vi "Periodic Tasks.vi"(8 "error in":errorcluster) -> ()   [LabVIEW 2017]
doc: "This VI runs in parallel to other tasks. It can contain as many user-defined periodic loops as you need. These can carry out PID or other sorts of timed response."
uses:
  Robot Global Data.vi
  <vilib>/Rock Robotics/WPI/ThirdParty/Phoenix-LabVIEW/Motor Controller/Controls/CTRE_Phoenix_MotorControl_ControlMode.ctl
  <vilib>/Rock Robotics/WPI/ThirdParty/Sensors/navX/_TypeDefs/FRIC_navX_DeviceNumbersTypeDef.ctl
  <vilib>/addons/control/pid/NI_PID_pid.lvlib
  <vilib>/Rock Robotics/WPI/ThirdParty/Phoenix-LabVIEW/Motor Controller/Get/CTRE_Phoenix_MotorController_GetQuadratureData.vi
  <vilib>/Rock Robotics/WPI/Solenoid/WPI_SolenoidValue.ctl
  Robust CSV/Robust CSV.lvlib
  Robust CSV/Write CSV File_2D.vi
  <vilib>/addons/control/pid/pid.llb/PID (DBL).vi
  <vilib>/Rock Robotics/WPI/Solenoid/WPI_SolenoidSetEnum.vi
panel:
  out "Loop Time":u32
  out "Right":cluster{dbl, i32}(graph)
  out "Left":T1(graph)
  out "clawUp":bool
  out "clawOpen":bool
  out "clawOut":bool
  out "clawIn":bool
  out "2slide":dbl
  out "1Sslide":dbl
  out "MotionProfilePos_Right":dbl
  out "MotionProfilePos_Left":dbl
  out "Right Pos Acutal":i32
  out "Left Pos Acutal":i32
  out "drive speed array":dbl[](array[numeric])
  out "Right Drive Speed":dbl
  out "Left Drive Speed":dbl
  out "output array":dbl[][](array[numeric])
  out "left 2":i32
  out "right 2":i32
  out "Yaw":dbl
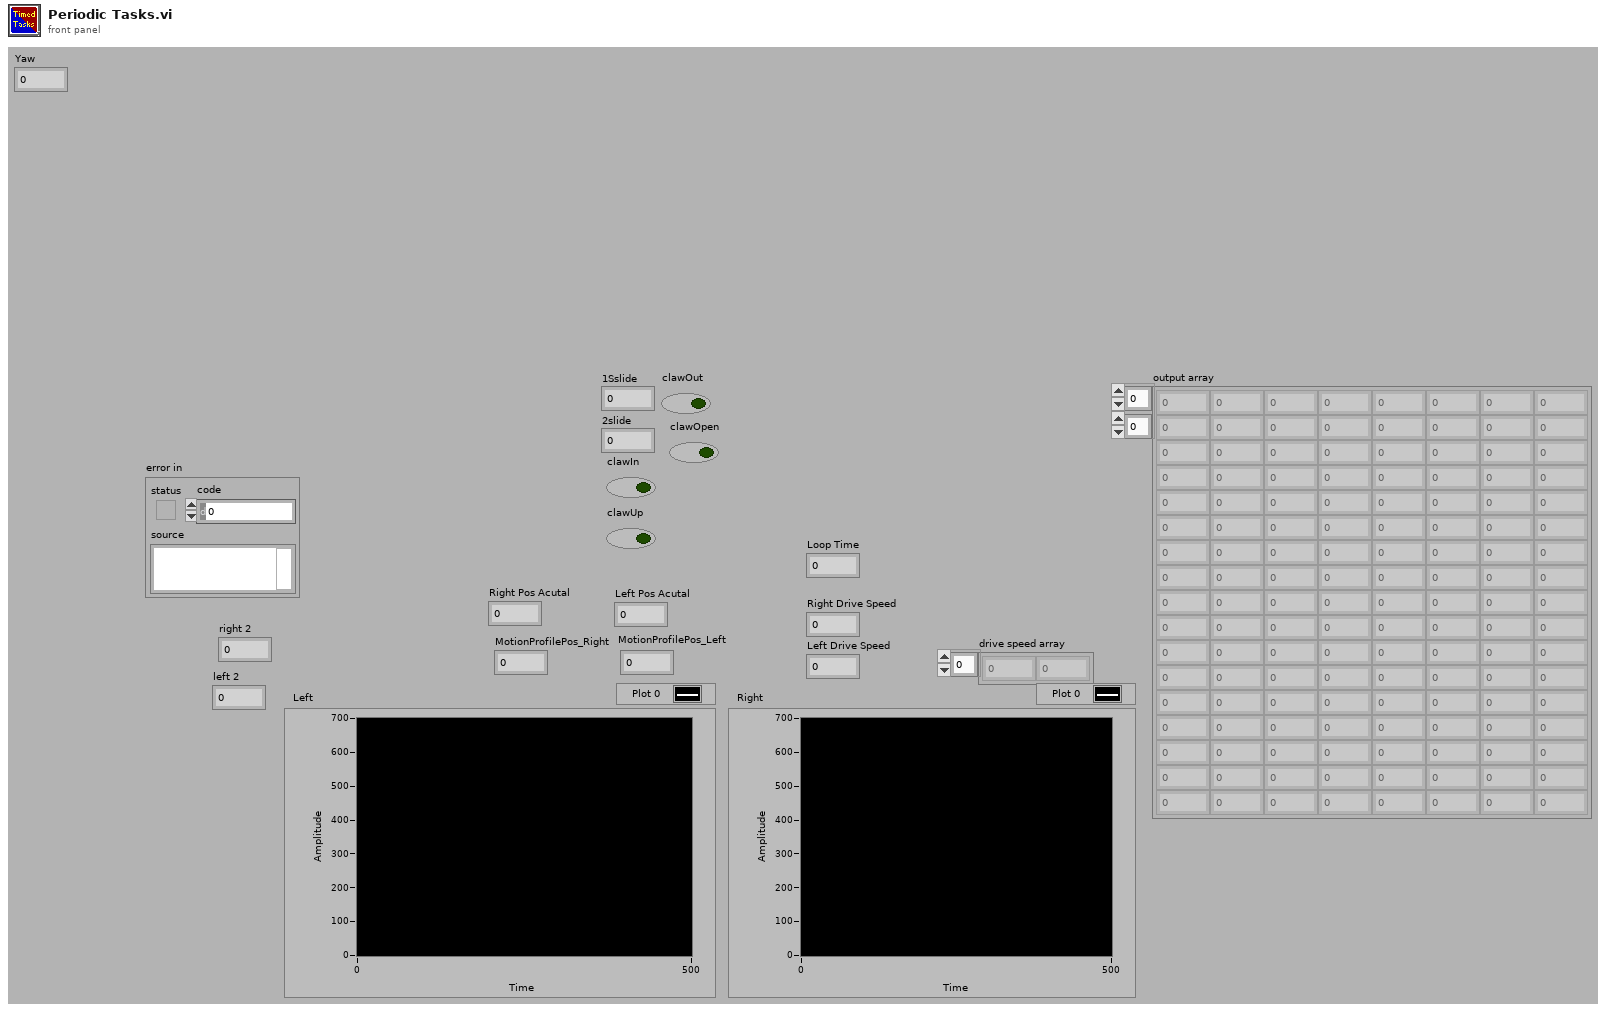
[diagram p1: front panel]
types:
  T1 = cluster{"MotionProfileVel_Right":dbl, "Quadrature Velocity":i32}
  T2 = typedef "WPI_MotorControlDeviceRef.ctl" = cluster{"DeviceStatus":errorcluster, "Type":T3, "PWM":cluster{"PWM Channel":T4, "DeadBand":T5}, "CAN":cluster{"Device Number":u8, "SetOutput VI Ref":variant, "GetOutput VI Ref":variant, "Enable VI Ref":variant, "Disable VI Ref":variant, "Data":variant}, "Invert":bool, "DIO PWM":cluster{"PWM \"Enable\" Channel":T4, "DIOChannel":T6, "PWM Rate":dbl}}
  T3 = typedef "WPI_MotorControlType.ctl" = enum16{"PWM", "CAN", "DIO PWM"}
  T4 = typedef "FPGA_DIOPWMChannel.ctl" = enum8{"PWM 0", "PWM 1", "PWM 2", "PWM 3", "PWM 4", "PWM 5", "PWM 6", "PWM 7", "PWM 8", "PWM 9", "PWM MXP 0", "PWM MXP 1", "PWM MXP 2", "PWM MXP 3", "PWM MXP 4", "PWM MXP 5", "PWM MXP 6", "PWM MXP 7", "PWM MXP 8", "PWM MXP 9", "Invalid"}
  T5 = typedef "WPI_PWMDeadband.ctl" = cluster{"Name":string, "maxPositivePwm":i32, "minPositivePwm":i32, "centerPwm":i32, "maxNegativePwm":i32, "minNegativePwm":i32, "angularRange":u16}
  T6 = typedef "FPGA_DIOChannel.ctl" = enum8{"DIO 0", "DIO 1", "DIO 2", "DIO 3", "DIO 4", "DIO 5", "DIO 6", "DIO 7", "DIO 8", "DIO 9", "DIO MXP 0", "DIO MXP 1", "DIO MXP 2", "DIO MXP 3", "DIO MXP 4", "DIO MXP 5", "DIO MXP 6", "DIO MXP 7", "DIO MXP 8", "DIO MXP 9", "DIO MXP 10", "DIO MXP 11", "DIO MXP 12", "DIO MXP 13", "DIO MXP 14", "DIO MXP 15", "SPI Port CS1", "SPI Port CS2", "SPI Port CS3", "SPI Port MISO", "SPI Port MOSI", "Invalid"}
  T7 = typedef "WPI_SolenoidDevRef.ctl" = cluster{"DevStatus":errorcluster, "Pneumatics Control Module":u8, "Forward Solenoid Channel":T8, "Reverse Solenoid Channel":T8}
  T8 = typedef "WPI_SolenoidChannel.ctl" = enum8{"Solenoid 0", "Solenoid 1", "Solenoid 2", "Solenoid 3", "Solenoid 4", "Solenoid 5", "Solenoid 6", "Solenoid 7", "Invalid"}
  T9 = typedef "WPI_SwitchDevRef.ctl" = cluster{"DevStatus":errorcluster, "DIO Channel":T6, "CntIndex":T10, "Normally Closed":bool}
  T10 = typedef "FPGA_CounterCtrSystemIndex.ctl" = enum8{"Ctr 0", "Ctr 1", "Ctr 2", "Ctr 3", "Ctr 4", "Ctr 5", "Ctr 6", "Ctr 7", "Invalid"}
  T11 = cluster{"proportional gain (Kc)":dbl, "integral time (Ti, min)":dbl, "derivative time (Td, min)":dbl}
  T12 = enum16{"Manual", "Turn For Angle", "Drive For Distance", "Motion Profile", "Recorded Auto File"}
  T13 = typedef "CTRE_Phoenix_MotorControl_ControlMode.ctl" = u16
  T14 = cluster{"MotionProfilePos_Right":dbl, "Quadrature Position":i32}
  T15 = typedef "WPI_SolenoidValue.ctl" = enum16{"Off", "On", "Forward", "Reverse"}
  T16 = typedef "FRIC_navX_DeviceNumbersTypeDef.ctl" = enum16{"Dev0", "Dev1", "Dev2", "Dev3"}
  T17 = cluster{"Yaw":dbl, "Roll":dbl, "Pitch":dbl, "Heading":dbl, "Fused Heading":dbl}
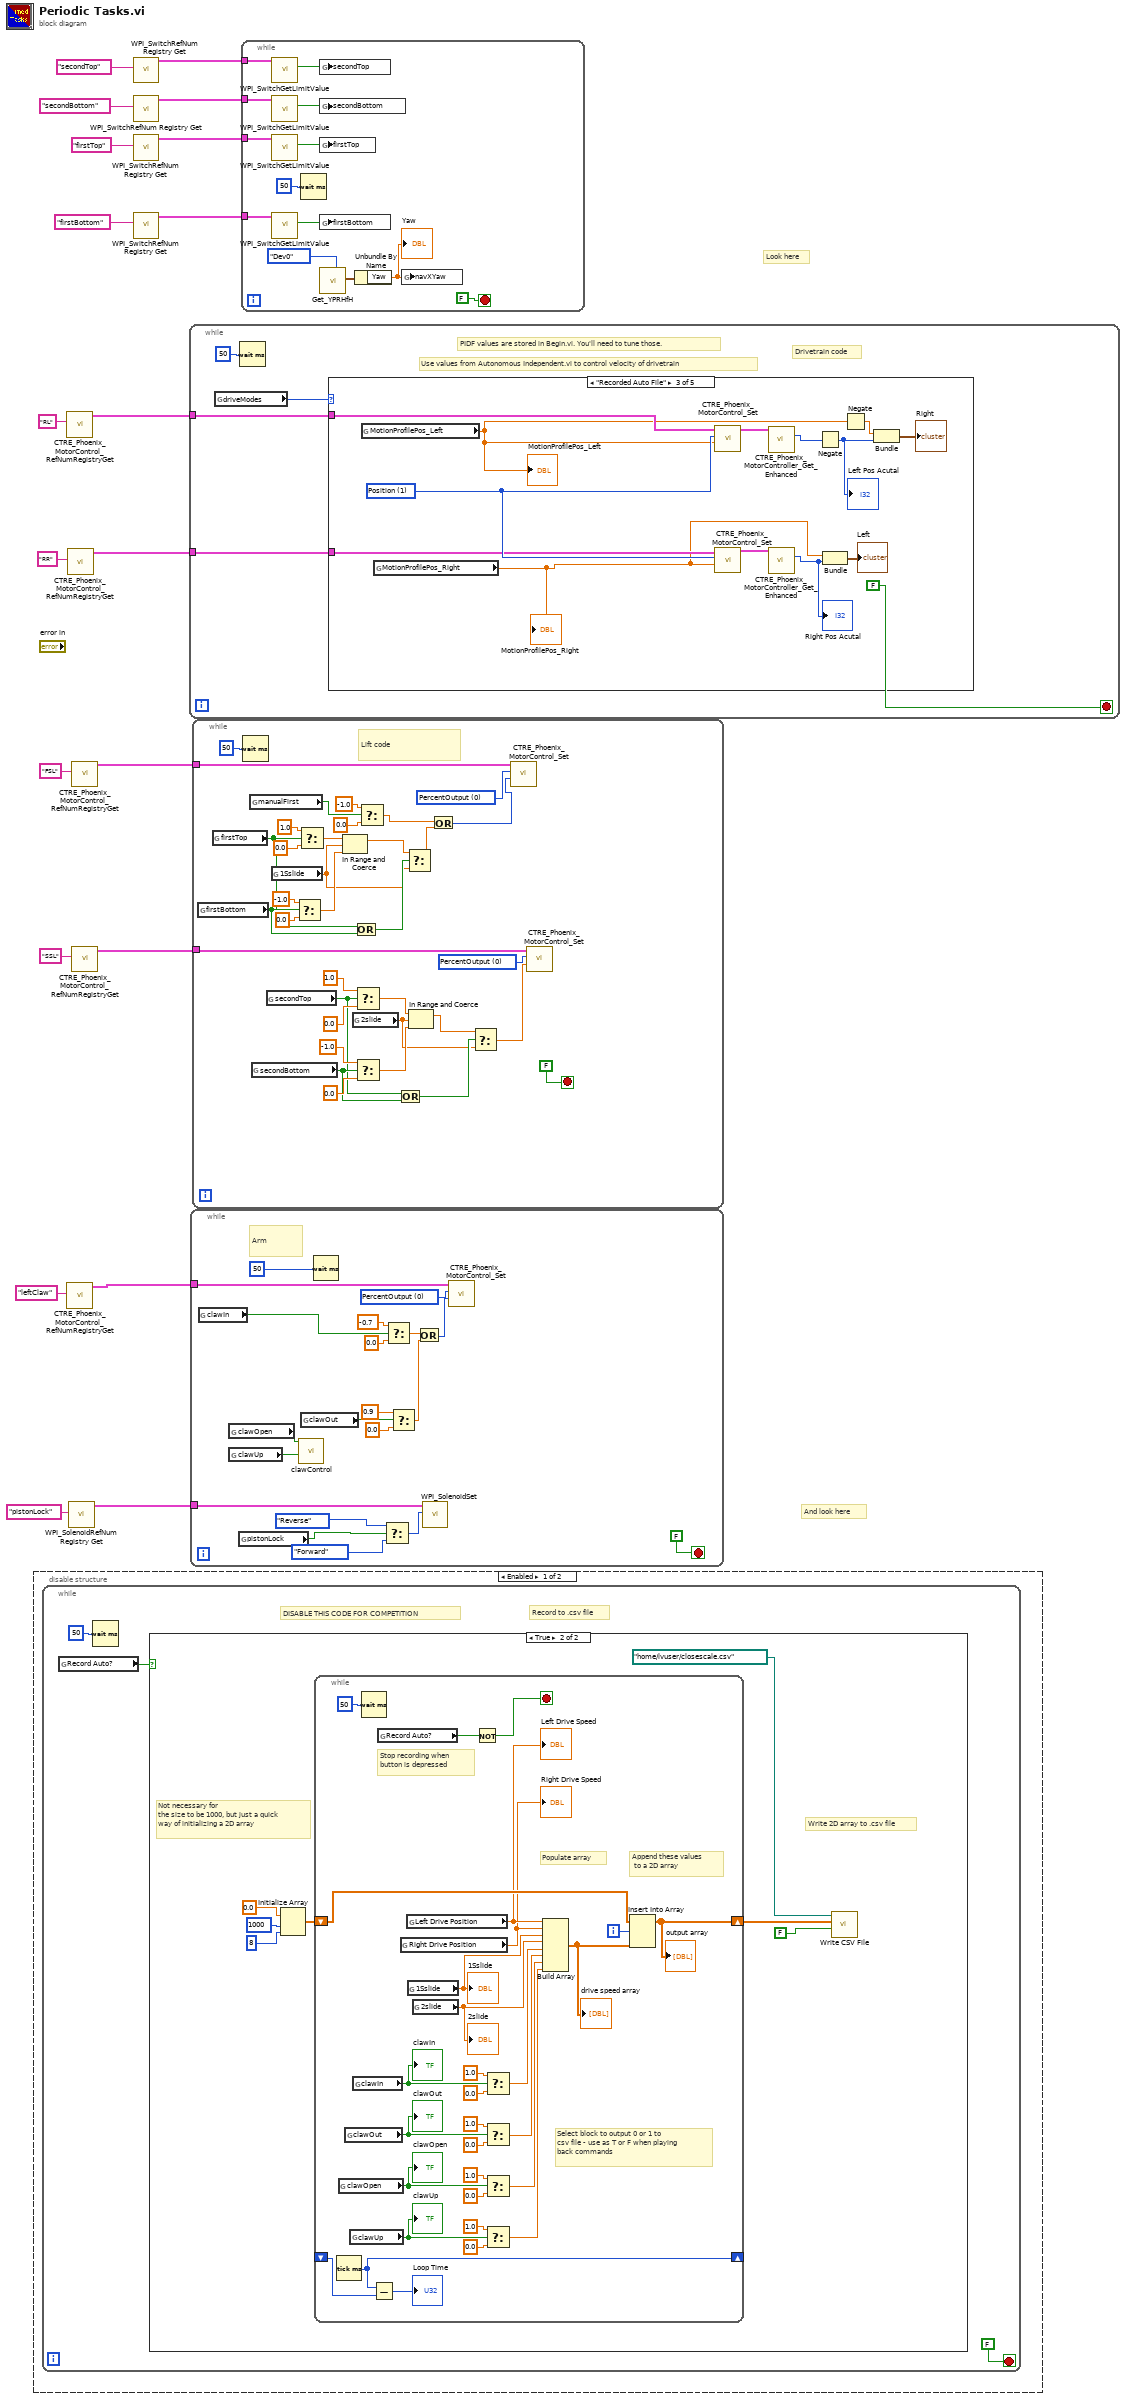
[diagram p0: block diagram]
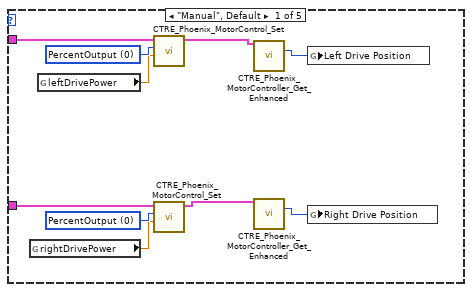
[diagram p4: hidden frame]
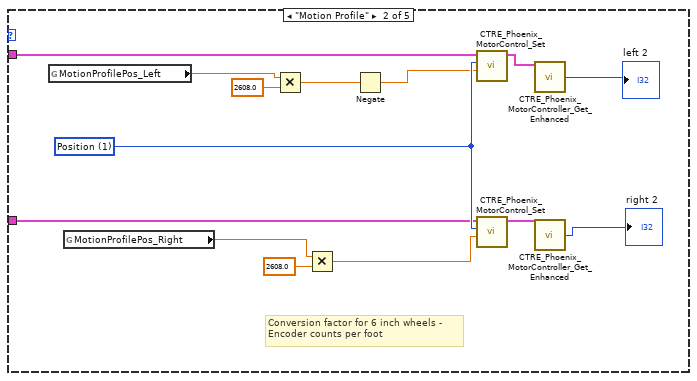
[diagram p5: hidden frame]
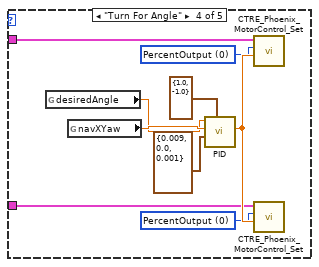
[diagram p6: hidden frame]
diagram:
  # "And look here"
  # "Look here"
  n1 = disable-structure shown="Enabled" {
    frame Enabled {
      n2 = while {
        stop <- FALSE stop-if-true
        # "Record to .csv file"
        # "DISABLE THIS CODE FOR COMPETITION"
        n3 = global read "Robot Global Data.vi" "Record Auto?"() -> (w22:bool)
        n4 = Wait (ms)(milliseconds to wait=u32 50) -> ()  [unwired: 1 out]
        n5 = case shown="True" w22 {
          frame False {
          }
          frame True {
            # "Not necessary for \nthe size to be 1000, but just a quick\nway of initializing a 2D array"
            # "Write 2D array to .csv file"
            n6 = Initialize Array(0.0 ("Left Drive Speed"), 1000 ("dimension size"), 8 ("dimension size")) -> (w27:dbl[][])
            n7 = while {
              shift-right: [w57] -> w24
              shift-left: w27 -> [w59]
              shift-right: [w32] -> _
              shift-left: _ -> [w33]
              i -> [w58]
              stop <- w56 stop-if-true
              # "Select block to output 0 or 1 to\ncsv file - use as T or F when playing\nback commands"
              # "Stop recording when \nbutton is depressed"
              # "Append these values\n to a 2D array"
              # "Populate array"
              n8 = Tick Count (ms)() -> (millisecond timer value=w32:u32)
              n9 = global read "Robot Global Data.vi" "clawOpen"() -> (w47:bool)
              "clawOpen" <- w47
              n10 = global read "Robot Global Data.vi" "clawOut"() -> (w48:bool)
              "clawOut" <- w48
              n11 = global read "Robot Global Data.vi" "clawUp"() -> (w46:bool)
              "clawUp" <- w46
              n12 = global read "Robot Global Data.vi" "clawIn"() -> (w49:bool)
              "clawIn" <- w49
              n13 = Wait (ms)(milliseconds to wait=u32 50) -> ()  [unwired: 1 out]
              n14 = Subtract(x=w32, y=w33) -> (x-y=→"Loop Time":u32)
              n15 = global read "Robot Global Data.vi" "Record Auto?"() -> (w52:bool)
              n16 = global read "Robot Global Data.vi" "Right Drive Position"() -> (w54:dbl)
              "Right Drive Speed" <- w54
              n17 = global read "Robot Global Data.vi" "Left Drive Position"() -> (w55:dbl)
              "Left Drive Speed" <- w55
              n18 = global read "Robot Global Data.vi" "1Sslide"() -> (w51:dbl)
              "1Sslide" <- w51
              n19 = global read "Robot Global Data.vi" "2slide"() -> (w50:dbl)
              "2slide" <- w50
              n20 = Not(x=w52) -> (.not. x?=w56:bool)
              n21 = Select(t=1.0, s=w49, f=0.0) -> (s? t:f=w37:dbl)
              n22 = Select(t=1.0, s=w48, f=0.0) -> (s? t:f=w36:dbl)
              n23 = Select(t=1.0, s=w47, f=0.0) -> (s? t:f=w35:dbl)
              n24 = Select(t=1.0, s=w46, f=0.0) -> (s? t:f=w34:dbl)
              n25 = Build Array(w55, w54, w51, w50, w37, w36, w35, w34) -> (w53:dbl[])
              "drive speed array" <- w53
              n26 = Insert Into Array(array=w59, index (row)=w58, new element=w53) -> (w57:dbl[][])  [unwired: 1 in]
              "output array" <- w57
            }
            n27 = call-poly "Write CSV File.vi"("append to file? (new file)"=FALSE, "Array"=w24, "file path in"=path "/home/lvuser/closescale.csv" ("file (use dialog)")) -> ()  [unwired: 7 in, 2 out]
          }
        }
      }
    }
    frame Disabled {
    }
  }
  n28 = call <vilib>:"CTRE_Phoenix_MotorControl_RefNumRegistryGet.vi"("refnum name"="RL") -> ("PhoenixMotorControlDevRef"=w3:T2)  [unwired: 9 in, 1 out]
  n29 = call <vilib>:"CTRE_Phoenix_MotorControl_RefNumRegistryGet.vi"("refnum name"="leftClaw") -> ("PhoenixMotorControlDevRef"=w7:T2)  [unwired: 9 in, 1 out]
  n30 = call <vilib>:"CTRE_Phoenix_MotorControl_RefNumRegistryGet.vi"("refnum name"="RR") -> ("PhoenixMotorControlDevRef"=w4:T2)  [unwired: 9 in, 1 out]
  n31 = call <vilib>:"WPI_SolenoidRefNum Registry Get.vi"("refnum name"="pistonLock") -> ("SolenoidDevRef"=w2:T7)  [unwired: 9 in, 1 out]
  n32 = call <vilib>:"CTRE_Phoenix_MotorControl_RefNumRegistryGet.vi"("refnum name"="FSL") -> ("PhoenixMotorControlDevRef"=w9:T2)  [unwired: 9 in, 1 out]
  n33 = call <vilib>:"CTRE_Phoenix_MotorControl_RefNumRegistryGet.vi"("refnum name"="SSL") -> ("PhoenixMotorControlDevRef"=w11:T2)  [unwired: 9 in, 1 out]
  n34 = call <vilib>:"WPI_SwitchRefNum Registry Get.vi"("refnum name"="secondTop") -> ("SwitchDevRef"=w15:T9)  [unwired: 9 in, 1 out]
  n35 = call <vilib>:"WPI_SwitchRefNum Registry Get.vi"("refnum name"="secondBottom") -> ("SwitchDevRef"=w16:T9)  [unwired: 9 in, 1 out]
  n36 = call <vilib>:"WPI_SwitchRefNum Registry Get.vi"("refnum name"="firstTop") -> ("SwitchDevRef"=w13:T9)  [unwired: 9 in, 1 out]
  n37 = call <vilib>:"WPI_SwitchRefNum Registry Get.vi"("refnum name"="firstBottom") -> ("SwitchDevRef"=w14:T9)  [unwired: 9 in, 1 out]
  n38 = while {
    tunnel: w4 -> [w62]
    tunnel: w3 -> [w61]
    stop <- FALSE stop-if-true
    # "Drivetrain code"
    # "PIDF values are stored in Begin.vi. You'll need to tune those."
    # "Use values from Autonomous Independent.vi to control velocity of drivetrain"
    n39 = global read "Robot Global Data.vi" "driveModes"() -> (w65:T12)
    n40 = Wait (ms)(milliseconds to wait=u32 50) -> ()  [unwired: 1 out]
    n41 = case shown="\"Recorded Auto File\"" w65 {
      tunnel: w62 -> [w71 w87 w100 w103 _]
      tunnel: w61 -> [w70 w88 w101 w104 _]
      frame "Manual", Default {
        w74 = T13 0 items=["PercentOutput"=0, "Position"=1, "Velocity"=2, "Current"=3, "Follower"=5, "MotionProfile"=6, "MotionMagic"=7, "MotionMagicArc"=8, "MotionProfileArc"=10, "Disabled"=15] ("Control Mode")
        w75 = T13 0 items=["PercentOutput"=0, "Position"=1, "Velocity"=2, "Current"=3, "Follower"=5, "MotionProfile"=6, "MotionMagic"=7, "MotionMagicArc"=8, "MotionProfileArc"=10, "Disabled"=15] ("Control Mode")
        n42 = global read "Robot Global Data.vi" "rightDrivePower"() -> (w72:dbl)
        n43 = global read "Robot Global Data.vi" "leftDrivePower"() -> (w73:dbl)
        n44 = call <vilib>:"CTRE_Phoenix_MotorControl_Set.vi"("Output"=w73, "Control Mode"=w74, "PhoenixMotorControlDevRef"=w70) -> ("PhoenixMotorControlDevRef"=w69:T2)  [unwired: 7 in, 1 out]
        n45 = call <vilib>:"CTRE_Phoenix_MotorControl_Set.vi"("Output"=w72, "Control Mode"=w75, "PhoenixMotorControlDevRef"=w71) -> ("PhoenixMotorControlDevRef"=w68:T2)  [unwired: 7 in, 1 out]
        n46 = call-poly <vilib>:"CTRE_Phoenix_MotorController_Get_Enhanced.vi"("PhoenixMotorControlDevRef"=w69) -> ("Quadrature Position"=w66:i32)  [unwired: 11 in, 3 out]
        n47 = call-poly <vilib>:"CTRE_Phoenix_MotorController_Get_Enhanced.vi"("PhoenixMotorControlDevRef"=w68) -> ("Quadrature Position"=w67:i32)  [unwired: 11 in, 3 out]
        n48 = global write "Robot Global Data.vi" "Left Drive Position"(w66) -> ()
        n49 = global write "Robot Global Data.vi" "Right Drive Position"(w67) -> ()
      }
      frame "Motion Profile" {
        w89 = T13 1 items=["PercentOutput"=0, "Position"=1, "Velocity"=2, "Current"=3, "Follower"=5, "MotionProfile"=6, "MotionMagic"=7, "MotionMagicArc"=8, "MotionProfileArc"=10, "Disabled"=15] ("Control Mode")
        # "Conversion factor for 6 inch wheels -\nEncoder counts per foot"
        n50 = global read "Robot Global Data.vi" "MotionProfilePos_Left"() -> (w81:dbl)
        n51 = global read "Robot Global Data.vi" "MotionProfilePos_Right"() -> (w77:dbl)
        n52 = Multiply(x=w81, y=2608.0) -> (x*y=w79:dbl)
        n53 = Multiply(x=w77, y=2608.0) -> (x*y=w76:dbl)
        n54 = Negate(x=w79) -> (-x=w82:dbl)
        n55 = call <vilib>:"CTRE_Phoenix_MotorControl_Set.vi"("Output"=w82, "Control Mode"=w89, "PhoenixMotorControlDevRef"=w88) -> ("PhoenixMotorControlDevRef"=w84:T2)  [unwired: 7 in, 1 out]
        n56 = call <vilib>:"CTRE_Phoenix_MotorControl_Set.vi"("Output"=w76, "Control Mode"=w89, "PhoenixMotorControlDevRef"=w87) -> ("PhoenixMotorControlDevRef"=w83:T2)  [unwired: 7 in, 1 out]
        n57 = call-poly <vilib>:"CTRE_Phoenix_MotorController_Get_Enhanced.vi"("PhoenixMotorControlDevRef"=w84) -> ("Quadrature Velocity"=→"left 2":i32)  [unwired: 11 in, 3 out]
        n58 = call-poly <vilib>:"CTRE_Phoenix_MotorController_Get_Enhanced.vi"("PhoenixMotorControlDevRef"=w83) -> ("Quadrature Velocity"=→"right 2":i32)  [unwired: 11 in, 3 out]
      }
      frame "Recorded Auto File" {
        w102 = T13 1 items=["PercentOutput"=0, "Position"=1, "Velocity"=2, "Current"=3, "Follower"=5, "MotionProfile"=6, "MotionMagic"=7, "MotionMagicArc"=8, "MotionProfileArc"=10, "Disabled"=15] ("Control Mode")
        n59 = global read "Robot Global Data.vi" "MotionProfilePos_Left"() -> (w94:dbl)
        "MotionProfilePos_Left" <- w94
        n60 = global read "Robot Global Data.vi" "MotionProfilePos_Right"() -> (w97:dbl)
        "MotionProfilePos_Right" <- w97
        n61 = call <vilib>:"CTRE_Phoenix_MotorControl_Set.vi"("Output"=w94, "Control Mode"=w102, "PhoenixMotorControlDevRef"=w101) -> ("PhoenixMotorControlDevRef"=w99:T2)  [unwired: 7 in, 1 out]
        n62 = call <vilib>:"CTRE_Phoenix_MotorControl_Set.vi"("Output"=w97, "Control Mode"=w102, "PhoenixMotorControlDevRef"=w100) -> ("PhoenixMotorControlDevRef"=w98:T2)  [unwired: 7 in, 1 out]
        n63 = call-poly <vilib>:"CTRE_Phoenix_MotorController_Get_Enhanced.vi"("PhoenixMotorControlDevRef"=w99) -> ("Quadrature Position"=w90:i32)  [unwired: 11 in, 3 out]
        n64 = call-poly <vilib>:"CTRE_Phoenix_MotorController_Get_Enhanced.vi"("PhoenixMotorControlDevRef"=w98) -> ("Quadrature Position"=w91:i32)  [unwired: 11 in, 3 out]
        "Right Pos Acutal" <- w91
        n65 = Negate(x=w90) -> (-x=w92:i32)
        "Left Pos Acutal" <- w92
        n66 = Bundle("MotionProfilePos_Right"=w97, "Quadrature Position"=w91) -> (→"Left":T14)  [unwired: 1 in]
        n67 = Negate(x=w94) -> (-x=w93:dbl)
        n68 = Bundle(w93, w92) -> (→"Right":cluster{dbl, i32})  [unwired: 1 in]
      }
      frame "Turn For Angle" {
        w108 = T13 0 items=["PercentOutput"=0, "Position"=1, "Velocity"=2, "Current"=3, "Follower"=5, "MotionProfile"=6, "MotionMagic"=7, "MotionMagicArc"=8, "MotionProfileArc"=10, "Disabled"=15] ("Control Mode")
        w107 = T13 0 items=["PercentOutput"=0, "Position"=1, "Velocity"=2, "Current"=3, "Follower"=5, "MotionProfile"=6, "MotionMagic"=7, "MotionMagicArc"=8, "MotionProfileArc"=10, "Disabled"=15] ("Control Mode")
        n69 = global read "Robot Global Data.vi" "desiredAngle"() -> (w105:dbl)
        n70 = global read "Robot Global Data.vi" "navXYaw"() -> (w106:dbl)
        n71 = call-poly <vilib>:"PID.vi"("output range"=cluster{"output high":dbl, "output low":dbl} {"output high"=1.0, "output low"=-1.0}, "PID gains"=T11 {"proportional gain (Kc)"=0.009, "integral time (Ti, min)"=0.0, "derivative time (Td, min)"=0.001}, "process variable"=w106, "setpoint"=w105) -> ("output"=w111:dbl)  [unwired: 6 in, 1 out]
        n72 = call <vilib>:"CTRE_Phoenix_MotorControl_Set.vi"("Output"=w111, "Control Mode"=w108, "PhoenixMotorControlDevRef"=w104) -> ()  [unwired: 7 in, 2 out]
        n73 = call <vilib>:"CTRE_Phoenix_MotorControl_Set.vi"("Output"=w111, "Control Mode"=w107, "PhoenixMotorControlDevRef"=w103) -> ()  [unwired: 7 in, 2 out]
      }
      frame "Drive For Distance" {
      }
    }
  }
  n74 = while {
    tunnel: w7 -> [w120]
    tunnel: w2 -> [w117]
    stop <- FALSE stop-if-true
    w121 = T13 0 items=["PercentOutput"=0, "Position"=1, "Velocity"=2, "Current"=3, "Follower"=5, "MotionProfile"=6, "MotionMagic"=7, "MotionMagicArc"=8, "MotionProfileArc"=10, "Disabled"=15] ("Control Mode")
    # "Arm"
    n75 = global read "Robot Global Data.vi" "clawIn"() -> (w112:bool)
    n76 = global read "Robot Global Data.vi" "clawOpen"() -> (w130:bool)
    n77 = global read "Robot Global Data.vi" "clawUp"() -> (w129:bool)
    n78 = global read "Robot Global Data.vi" "pistonLock"() -> (w114:bool)
    n79 = call "clawControl.vi"("open"=w129, "up"=w130) -> ()  [unwired: 10 in]
    n80 = global read "Robot Global Data.vi" "clawOut"() -> (w125:bool)
    n81 = Wait (ms)(milliseconds to wait=u32 50) -> ()  [unwired: 1 out]
    n82 = Select(t=WPI_SolenoidValue."Reverse" ("Value"), s=w114, f=WPI_SolenoidValue."Forward") -> (s? t:f=w113:T15)
    n83 = Select(t=-0.7, s=w112, f=0.0) -> (s? t:f=w126:dbl)
    n84 = Select(t=0.9, s=w125, f=0.0) -> (s? t:f=w127:dbl)
    n85 = Or(x=w126, y=w127) -> (x .or. y?=w128:i32)
    n86 = call-poly <vilib>:"WPI_SolenoidSet.vi"("Value"=w113, "SolenoidDevRef"=w117) -> ()  [unwired: 8 in, 2 out]
    n87 = call <vilib>:"CTRE_Phoenix_MotorControl_Set.vi"("Output"=w128, "Control Mode"=w121, "PhoenixMotorControlDevRef"=w120) -> ()  [unwired: 7 in, 2 out]
  }
  n88 = while {
    tunnel: w11 -> [w148]
    tunnel: w9 -> [w147]
    stop <- FALSE stop-if-true
    w164 = T13 0 items=["PercentOutput"=0, "Position"=1, "Velocity"=2, "Current"=3, "Follower"=5, "MotionProfile"=6, "MotionMagic"=7, "MotionMagicArc"=8, "MotionProfileArc"=10, "Disabled"=15] ("Control Mode")
    w165 = T13 0 items=["PercentOutput"=0, "Position"=1, "Velocity"=2, "Current"=3, "Follower"=5, "MotionProfile"=6, "MotionMagic"=7, "MotionMagicArc"=8, "MotionProfileArc"=10, "Disabled"=15] ("Control Mode")
    # "Lift code"
    n89 = global read "Robot Global Data.vi" "firstBottom"() -> (w144:bool)
    n90 = global read "Robot Global Data.vi" "firstTop"() -> (w143:bool)
    n91 = Wait (ms)(milliseconds to wait=u32 50) -> ()  [unwired: 1 out]
    n92 = global read "Robot Global Data.vi" "manualFirst"() -> (w151:bool)
    n93 = global read "Robot Global Data.vi" "secondBottom"() -> (w137:bool)
    n94 = global read "Robot Global Data.vi" "secondTop"() -> (w136:bool)
    n95 = global read "Robot Global Data.vi" "1Sslide"() -> (w141:dbl)
    n96 = Select(t=-1.0, s=w144, f=0.0) -> (s? t:f=w163:dbl)
    n97 = Select(t=1.0, s=w143, f=0.0) -> (s? t:f=w162:dbl)
    n98 = In Range and Coerce(upper limit=w162, x=w141, lower limit=w163) -> (coerced(x)=w145:dbl)  [unwired: 1 out]
    n99 = global read "Robot Global Data.vi" "2slide"() -> (w134:dbl)
    n100 = Or(x=w143, y=w144) -> (x .or. y?=w142:bool)
    n101 = Select(t=1.0, s=w136, f=0.0) -> (s? t:f=w153:dbl)
    n102 = Select(t=-1.0, s=w137, f=0.0) -> (s? t:f=w152:dbl)
    n103 = Select(t=-1.0, s=w151, f=0.0) -> (s? t:f=w139:dbl)
    n104 = Or(x=w136, y=w137) -> (x .or. y?=w135:bool)
    n105 = Select(t=w145, s=w142, f=w141) -> (s? t:f=w140:dbl)
    n106 = In Range and Coerce(upper limit=w153, x=w134, lower limit=w152) -> (coerced(x)=w133:dbl)  [unwired: 1 out]
    n107 = Or(x=w139, y=w140) -> (x .or. y?=w138:i32)
    n108 = Select(t=w133, s=w135, f=w134) -> (s? t:f=w132:dbl)
    n109 = call <vilib>:"CTRE_Phoenix_MotorControl_Set.vi"("Output"=w138, "Control Mode"=w164, "PhoenixMotorControlDevRef"=w147) -> ()  [unwired: 7 in, 2 out]
    n110 = call <vilib>:"CTRE_Phoenix_MotorControl_Set.vi"("Output"=w132, "Control Mode"=w165, "PhoenixMotorControlDevRef"=w148) -> ()  [unwired: 7 in, 2 out]
  }
  n111 = while {
    tunnel: w16 -> [w170]
    tunnel: w15 -> [w169]
    tunnel: w14 -> [w168]
    tunnel: w13 -> [w167]
    stop <- FALSE stop-if-true
    n112 = call <vilib>:"WPI_SwitchGetLimitValue.vi"("SwitchDevRef"=w169) -> ("Switch Pressed"=w176:bool)  [unwired: 8 in, 2 out]
    n113 = call <vilib>:"WPI_SwitchGetLimitValue.vi"("SwitchDevRef"=w170) -> ("Switch Pressed"=w175:bool)  [unwired: 8 in, 2 out]
    n114 = call <vilib>:"WPI_SwitchGetLimitValue.vi"("SwitchDevRef"=w167) -> ("Switch Pressed"=w177:bool)  [unwired: 8 in, 2 out]
    n115 = call <vilib>:"WPI_SwitchGetLimitValue.vi"("SwitchDevRef"=w168) -> ("Switch Pressed"=w178:bool)  [unwired: 8 in, 2 out]
    n116 = Wait (ms)(milliseconds to wait=u32 50) -> ()  [unwired: 1 out]
    n117 = global write "Robot Global Data.vi" "secondTop"(w176) -> ()
    n118 = global write "Robot Global Data.vi" "secondBottom"(w175) -> ()
    n119 = global write "Robot Global Data.vi" "firstTop"(w177) -> ()
    n120 = global write "Robot Global Data.vi" "firstBottom"(w178) -> ()
    n121 = call <vilib>:"Get_YPRHfH.vi"("Device Number"=FRIC_navX_DeviceNumbersTypeDef."Dev0") -> ("YRPHfH"=w172:T17)  [unwired: 10 in]
    n122 = Unbundle By Name(w172) -> ("Yaw"=w171:dbl)
    "Yaw" <- w171
    n123 = global write "Robot Global Data.vi" "navXYaw"(w171) -> ()
  }
